vi "xio.tmpdir_lua.vi"(5 "LuaVIEW reference":T1) -> (15 "error out":errorcluster)   [LabVIEW 2012]
doc: "Returns the path to the temporary directory.\nResults:\nstr:path"
uses:
  typedefs/t_LuaVIEW Reference.ctl
  subvis/private/LuaVIEW Push (path).vi
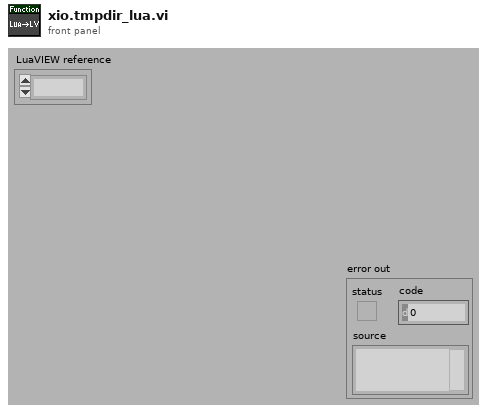
[diagram p1: front panel]
types:
  T1 = typedef "t_LuaVIEW Reference.ctl" = refnum<k1>
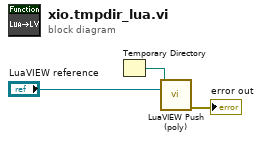
[diagram p0: block diagram]
diagram:
  n1 = Temporary Directory() -> (w1:path)
  n2 = call-poly "LuaVIEW Push (poly).vi"("path"=w1, "LuaVIEW reference in"="LuaVIEW reference") -> ("error out"=→"error out":errorcluster)  [unwired: 12 in, 1 out]
